vi "Spectrograph_monitorCommand_start.vi"(8 "error in (no error)":errorcluster, 11 "command_start_Ctl":T1) -> (0 "error out":errorcluster, 2 "function return":i32, 3 "command_start_Ctl out":T1)   [LabVIEW 2016, in "SALLV_Spectrograph.lvlib"]
doc: "int Spectrograph_shm_monitorCommand_startLV(Spectrograph_command_startLV *command_start_Ctl );"
uses:
  SALLV_Spectrograph.lvlib
  DataTypes/command_start.ctl
  SALLV_Spectrograph.so
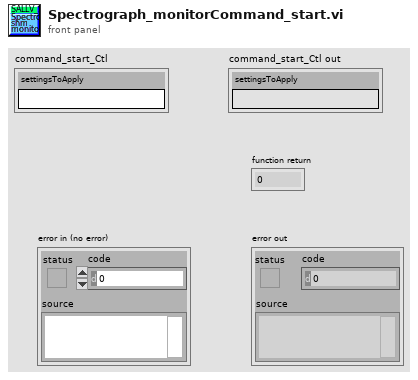
[diagram p1: front panel]
types:
  T1 = typedef "SALLV_Spectrograph.lvlib/command_start.ctl" = cluster{"settingsToApply":string}
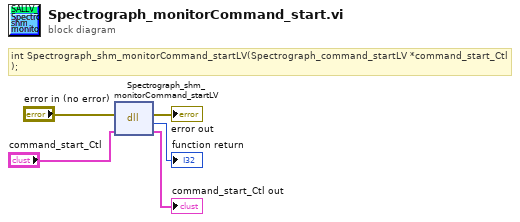
[diagram p0: block diagram]
diagram:
  # "int Spectrograph_shm_monitorCommand_startLV(Spectrograph_command_startLV *command_start_Ctl );"
  n1 = dll-call lib="home/harini/TCS/SALLV_Spectrograph/SALLV_Spectrograph.*" fn="Spectrograph_shm_monitorCommand_startLV"(error in="error in (no error)", "command_start_Ctl"="command_start_Ctl") -> (error out=→"error out":errorcluster, →"function return":i32, "command_start_Ctl"=→"command_start_Ctl out":T1)  [unwired: 2 in, 1 out]
